vi "Set Parameter.vi"(8 "error in (no error)":errorcluster, 10 "Parameter":refnum<class "AbstractData.lvclass">, 11 "ParameterDevice in":refnum<class "ParameterDevice.lvclass">) -> (0 "error out":errorcluster, 3 "ParameterDevice out":refnum<class "ParameterDevice.lvclass">)   [LabVIEW 2014, in "ParameterDevice.lvclass"]
uses:
  ParameterDevice.lvclass
  Model/Data/AbstractData/AbstractData.lvclass
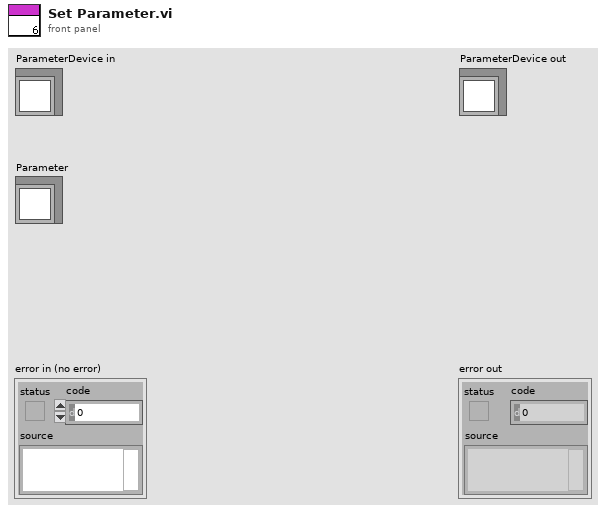
[diagram p1: front panel]
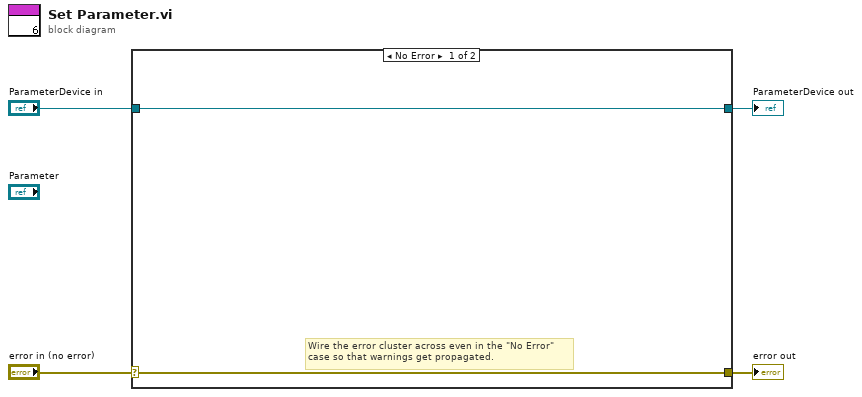
[diagram p0: block diagram]
diagram:
  n1 = case shown="No Error" "error in (no error)" {
    selector: "error in (no error)" -> [w5 w8]
    tunnel: [w5 w8] -> w3
    tunnel: [w6 w7] -> w1
    tunnel: "ParameterDevice in" -> [w6 w7]
    frame No Error {
      # "Wire the error cluster across even in the \"No Error\"\ncase so that warnings get propagated."
    }
    frame Error {
    }
  }
  "error out" <- w3
  "ParameterDevice out" <- w1
